vi "WILT Find Specific Label Name.vi"(10 "Search Label Name":string="Water Valve", 11 "Agilent Channels Raw":T1[](array[typedef])) -> (3 "Specific":T1[](array[typedef]))   [LabVIEW 2016]
uses:
  Type Definitions/WILT Agilent Channel Definition.ctl
  <vilib>/Utility/error.llb/whitespace.ctl
panel:
  out "Numeric":i32
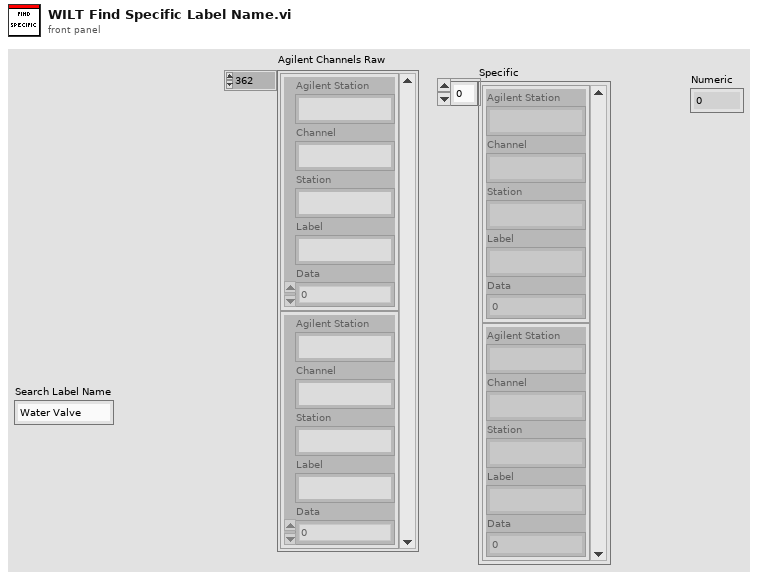
[diagram p1: front panel]
types:
  T1 = typedef "WILT Agilent Channel Definition.ctl" = cluster{"Channel":string, "Station":string, "Label":string, "Agilent Station":string, "Data":dbl}
  T2 = typedef "whitespace.ctl" = u16
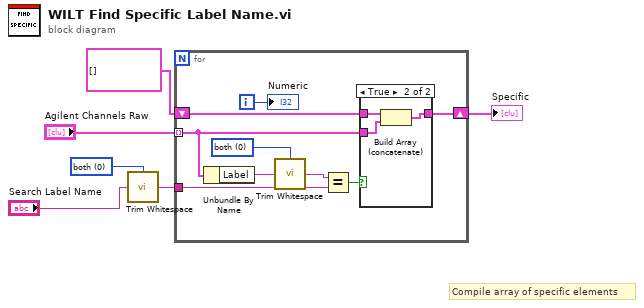
[diagram p0: block diagram]
diagram:
  w1 = T2 0 items=["both", "start of string", "end of string"] ("location (both)")
  # "Compile array of specific elements"
  n1 = call <vilib>:"Trim Whitespace.vi"("string"="Search Label Name", "location (both)"=w1) -> ("trimmed string"=w2:string)
  n2 = for {
    tunnel: "Agilent Channels Raw" -> [w12] mode=indexing
    shift-right: [w13] -> w6
    shift-left: T1[] [] -> [w14]
    tunnel: w2 -> [w11]
    i -> [w8]
    w9 = T2 0 items=["both", "start of string", "end of string"] ("location (both)")
    n3 = Unbundle By Name(w12) -> ("Label"=w7:string)
    n4 = call <vilib>:"Trim Whitespace.vi"("string"=w7, "location (both)"=w9) -> ("trimmed string"=w10:string)
    n5 = Equal?(x=w10, y=w11) -> (x = y?=w15:bool)
    n6 = case shown="True" w15 {
      tunnel: w12 -> [_ w17]
      tunnel: w14 -> [w16 w19]
      tunnel: [w16 w18] -> w13
      frame False {
      }
      frame True {
        n7 = Build Array (concatenate)(w19, w17) -> (w18:T1[])
      }
    }
    "Numeric" <- w8
  }
  "Specific" <- w6
